vi "Convert Joystick Axis Event Data.vi"(11 "Event Data":u8[](array[numeric]) format="%.0x") -> (3 "Joystick Axis Event":T1 {"Padding 4" format="%.0x"; "Value" format="%.0x"; "Padding 3" format="%.0x"; "Padding 2" format="%.0x"; "Which" format="%.0x"; "Type" format="%.0x"})   [LabVIEW 2015, in "LibSDL2.lvlib"]
uses:
  LibSDL2.lvlib
  Controls/Joysitck Axis Event.ctl
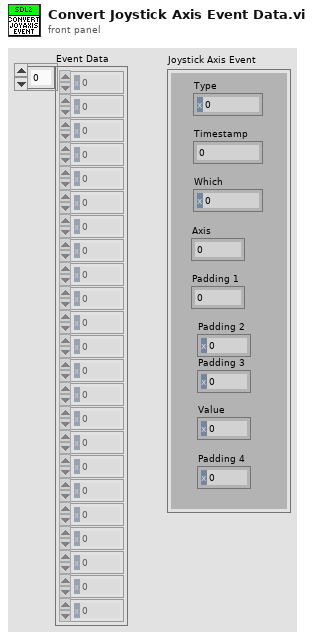
[diagram p1: front panel]
types:
  T1 = typedef "LibSDL2.lvlib/Joysitck Axis Event.ctl" = cluster{"Type":u32, "Timestamp":u32, "Which":i32, "Axis":u8, "Padding 1":u8, "Padding 2":u8, "Padding 3":u8, "Value":i16, "Padding 4":u16}
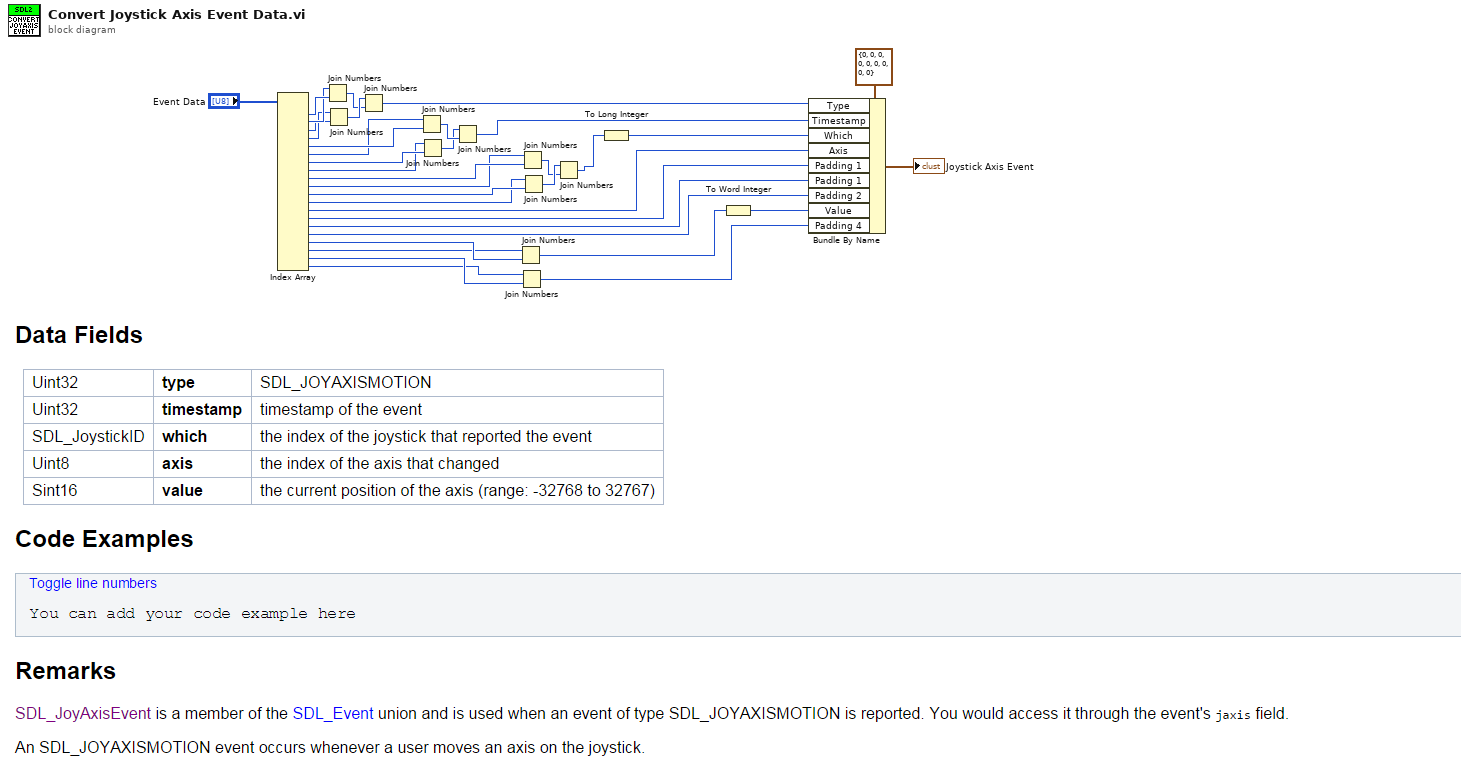
[diagram p0: block diagram]
diagram:
  n1 = Index Array(array="Event Data") -> (element #1=w34:u8, element #2=w33:u8, element #3=w31:u8, element #4=w32:u8, element #5=w25:u8, element #6=w24:u8, element #7=w23:u8, element #8=w22:u8, element #9=w18:u8, element #10=w17:u8, element #11=w16:u8, element #12=w15:u8, element #13=w14:u8, element #14=w13:u8, element #15=w12:u8, element #16=w11:u8, element #17=w10:u8, element #18=w9:u8, element #19=w8:u8, element #20=w7:u8)  [unwired: 20 in]
  n2 = Join Numbers(hi=w33, lo=w34) -> ((hi.lo)=w29:u16)
  n3 = Join Numbers(hi=w32, lo=w31) -> ((hi.lo)=w30:u16)
  n4 = Join Numbers(hi=w30, lo=w29) -> ((hi.lo)=w28:u32)
  n5 = Join Numbers(hi=w24, lo=w25) -> ((hi.lo)=w27:u16)
  n6 = Join Numbers(hi=w22, lo=w23) -> ((hi.lo)=w26:u16)
  n7 = Join Numbers(hi=w26, lo=w27) -> ((hi.lo)=w21:u32)
  n8 = Join Numbers(hi=w9, lo=w10) -> ((hi.lo)=w4:u16)
  n9 = Join Numbers(hi=w7, lo=w8) -> ((hi.lo)=w2:u16)
  n10 = Join Numbers(hi=w17, lo=w18) -> ((hi.lo)=w19:u16)
  n11 = Join Numbers(hi=w15, lo=w16) -> ((hi.lo)=w20:u16)
  n12 = Join Numbers(hi=w20, lo=w19) -> ((hi.lo)=w6:u32)
  n13 = To Long Integer(number=w6) -> (32bit integer=w5:i32)
  n14 = To Word Integer(number=w4) -> (16bit integer=w3:i16)
  n15 = Bundle By Name(cluster=T1 {"Type"=0, "Timestamp"=0, "Which"=0, "Axis"=0, "Padding 1"=0, "Padding 2"=0, "Padding 3"=0, "Value"=0, "Padding 4"=0} ("Joystick Axis Event"), "Type"=w28, "Timestamp"=w21, "Which"=w5, "Axis"=w14, "Padding 1"=w13, "Padding 1"=w12, "Padding 2"=w11, "Value"=w3, "Padding 4"=w2) -> (→"Joystick Axis Event":T1)
